vi "Read BufSize.vi"(8 "error in (no error)":errorcluster, 11 "DAQ Task in":refnum<class "DAQ Task.lvclass">) -> (0 "error out":errorcluster, 2 "BufSize":u32, 3 "DAQ Task out":refnum<class "DAQ Task.lvclass">)   [LabVIEW 2012, in "Data Acquisition.lvlib" / "DAQ Task.lvclass"]
uses:
  DAQ Task.lvclass
  DAQ Task.lvclass/DAQ Task.ctl
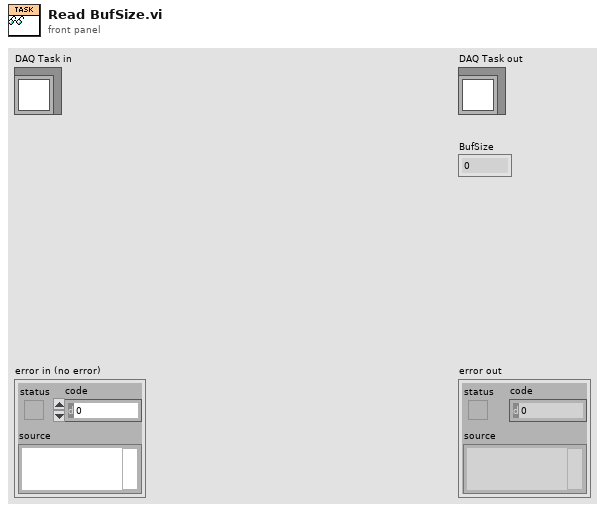
[diagram p1: front panel]
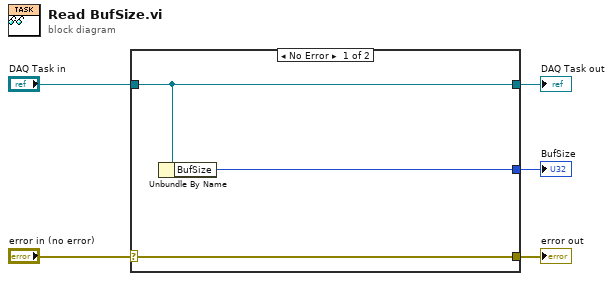
[diagram p0: block diagram]
diagram:
  n1 = case shown="No Error" "error in (no error)" {
    selector: "error in (no error)" -> [w8 w9]
    tunnel: [w8 w9] -> w4
    tunnel: [w7 w10] -> w2
    tunnel: "DAQ Task in" -> [w7 w10]
    tunnel: [w6 _] -> w1
    frame No Error {
      n2 = Unbundle By Name(w7) -> ("BufSize"=w6:u32)
    }
    frame Error {
    }
  }
  "error out" <- w4
  "DAQ Task out" <- w2
  "BufSize" <- w1
